vi "GetPosition.vi"() -> (2 "Y":dbl, 3 "X":dbl)   [LabVIEW 2014]
uses:
  c_Query_States.ctl
  c_InstructionEnum.ctl
  g_CommandParam.vi
  g_ECS02_Command.vi
panel:
  out "Query Response":string
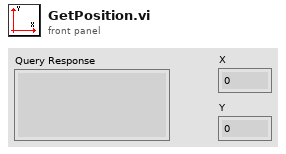
[diagram p1: front panel]
types:
  T1 = typedef "c_Query_States.ctl" = enum16{"Send Query", "Get Response ", "Get Position", "Get Ready Status"}
  T2 = typedef "c_InstructionEnum.ctl" = enum16{"Move Absolute", "Increment", "Move Home", "Motion Kill", "Move Plate", "Set Stepsize", "Query Position"}
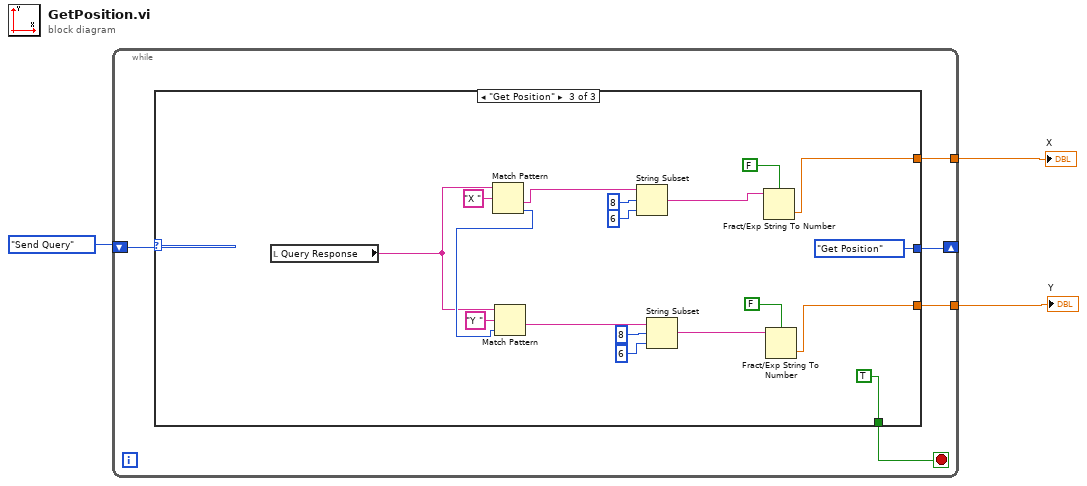
[diagram p0: block diagram]
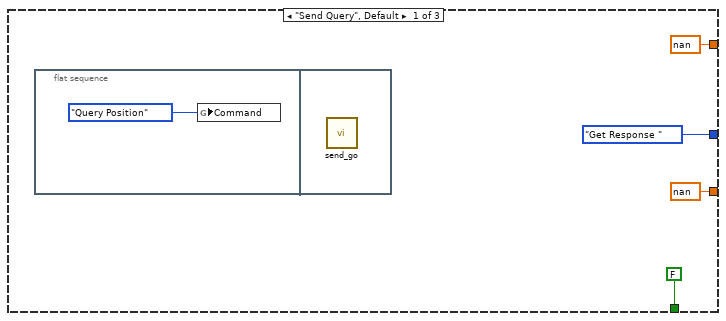
[diagram p2: hidden frame]
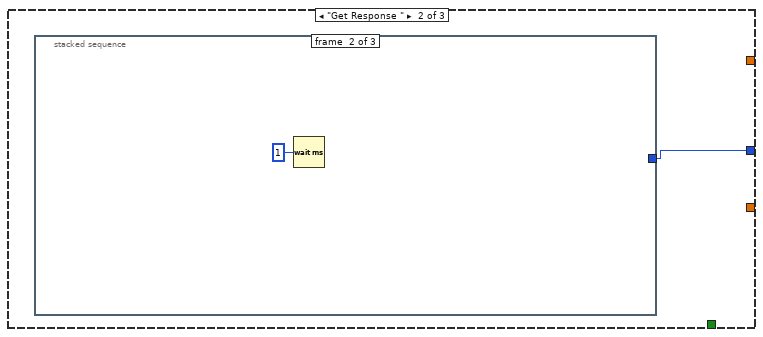
[diagram p3: hidden frame]
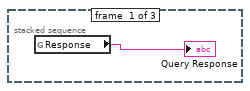
[diagram p4: hidden frame]
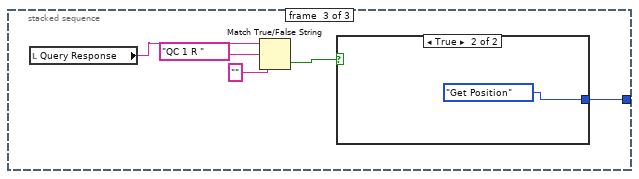
[diagram p5: hidden frame]
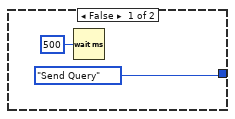
[diagram p6: hidden frame]
diagram:
  n1 = while {
    shift-right: [w7] -> _
    shift-left: c_Query_States."Send Query" -> [w8]
    tunnel: [w6] -> w2
    tunnel: [w5] -> w1
    stop <- w4 stop-if-true
    n2 = case shown="\"Get Position\"" w8 {
      tunnel: [c_Query_States."Get Response " w14 c_Query_States."Get Position"] -> w7
      tunnel: [nan _ w28] -> w6
      tunnel: [nan _ w27] -> w5
      tunnel: [FALSE _ TRUE] -> w4
      frame "Send Query", Default {
        n3 = flat-sequence {
          frame #0 {
            n4 = global write "g_CommandParam.vi" "Command"(c_InstructionEnum."Query Position" ("Command")) -> ()
          }
          frame #1 {
            n5 = call "send_go.vi"() -> ()  [unwired: 12 in]
          }
        }
      }
      frame "Get Response " {
        n6 = stacked-sequence {
          tunnel: [_ _ w19] -> w14
          frame #0 {
            n7 = global read "g_ECS02_Command.vi" "Response"() -> (→"Query Response":string)
          }
          frame #1 {
            n8 = Wait (ms)(milliseconds to wait=u32 1) -> ()  [unwired: 1 out]
          }
          frame #2 {
            n9 = local read "Query Response"() -> (w18:string)
            n10 = Match True/False String(2:"" ("false string"), 3:"QC 1 R " ("true string"), 4:w18) -> (0:w17:bool)  [unwired: 1 out]
            n11 = case shown="True" w17 {
              tunnel: [c_Query_States."Send Query" c_Query_States."Get Position"] -> w19
              frame False {
                n12 = Wait (ms)(milliseconds to wait=u32 500) -> ()  [unwired: 1 out]
              }
              frame True {
              }
            }
          }
        }
      }
      frame "Get Position" {
        n13 = local read "Query Response"() -> (w29:string)
        n14 = Match Pattern(string=w29, regular expression="X ") -> (after substring=w40:string, offset past match=w36:i32)  [unwired: 1 in, 2 out]
        n15 = Match Pattern(string=w29, regular expression="Y ", offset (0)=w36) -> (after substring=w39:string)  [unwired: 3 out]
        n16 = String Subset(string=w40, offset (0)=8, length (rest)=6 ("length (rest)")) -> (substring=w30:string)
        n17 = String Subset(string=w39, offset (0)=8, length (rest)=6 ("length (rest)")) -> (substring=w32:string)
        n18 = Fract/Exp String To Number(use system decimal point (T)=FALSE, string=w30) -> (number=w27:dbl)  [unwired: 2 in, 1 out]
        n19 = Fract/Exp String To Number(use system decimal point (T)=FALSE, string=w32) -> (number=w28:dbl)  [unwired: 2 in, 1 out]
      }
    }
  }
  "X" <- w1
  "Y" <- w2
